vi "UTF-8 to Text Wrapper.vi"(8 "error in":errorcluster, 10 "encoding (system default=-1)":i32=-1, 11 "utf-8 text":string) -> (0 "error out":errorcluster, 3 "text":string)   [LabVIEW 2022 SP3, in "hse-misc.lvlib"]
doc: "Converts UTF-8 text to text encoded in the specified system.\n\n____\nHAMPEL SOFTWARE ENGINEERING v3.8.0 (2023-12-18 14:41)"
uses:
  hse-misc.lvlib
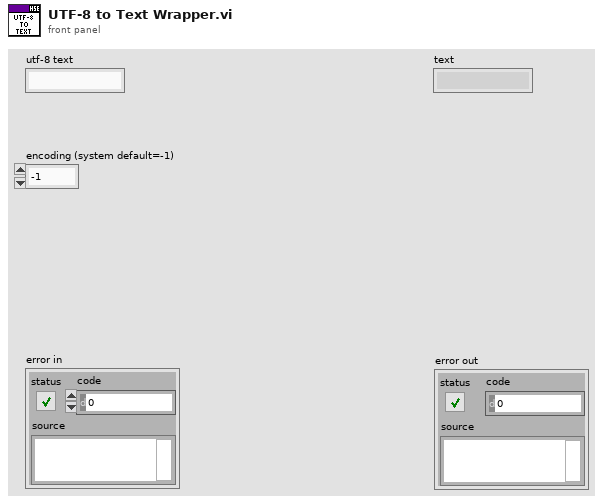
[diagram p1: front panel]
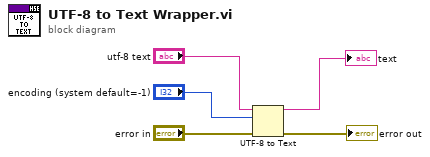
[diagram p0: block diagram]
diagram:
  n1 = UTF-8 to Text(8:"error in", 10:"encoding (system default=-1)", 11:"utf-8 text") -> (0:→"error out":errorcluster, 3:→"text":string)
